vi "Unscale 32 Bit.vi"(8 "error in (no error)":errorcluster, 11 "Data Scaling in":refnum<class "Data Scaling.lvclass">) -> (0 "error out":errorcluster, 3 "Data Scaling out":refnum<class "Data Scaling.lvclass">)   [LabVIEW 2020, in "Unit Tests.lvlib" / "Data Scaling.lvclass"]
uses:
  Data Scaling.lvclass
  Frames & Messages/TypeDefs/Scaling Information.ctl
  <vilib>/addons/_JKI Toolkits/Caraya/classes/Test/Test.lvclass
  <vilib>/addons/_JKI Toolkits/Caraya/classes/Assert/Assert.lvclass
  BCI-1553 API.lvlib
panel:
  out "unscaled number":u64 format="%064b"
  out "base number":u64 format="%064b"
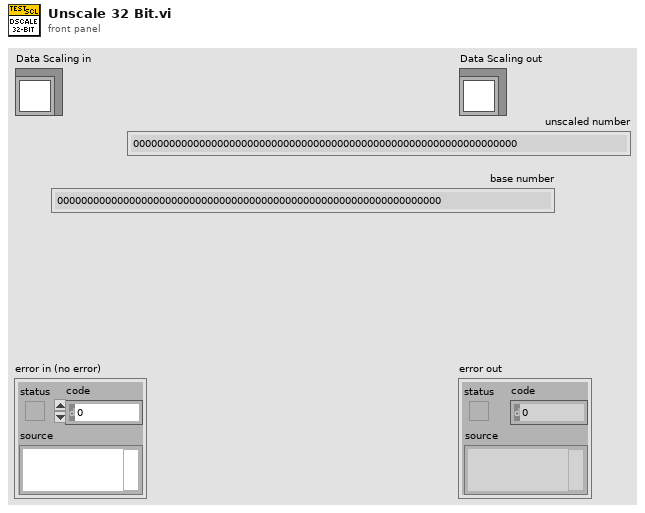
[diagram p1: front panel]
types:
  T1 = typedef "BCI-1553 API.lvlib/Scaling Information.ctl" = cluster{"Bit Offset":i32, "Bit Count":i32, "LSB Resolution":dbl, "2's Complement":bool, "Big Endian":bool, "Sign Bit":bool}
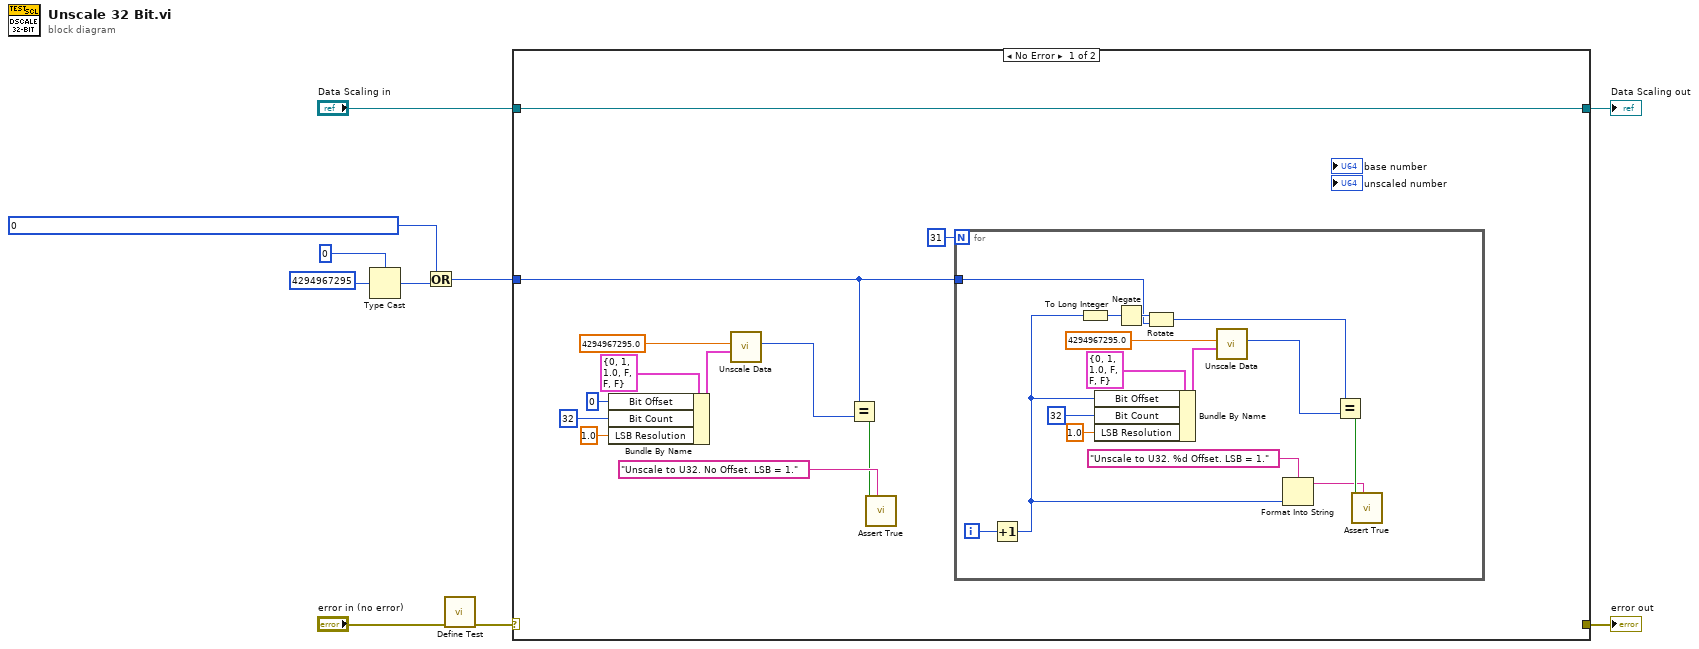
[diagram p0: block diagram]
diagram:
  n1 = Type Cast(type=u64 0 ("x"), x=u32 4294967295 ("unsigned 8bit integer")) -> (*(type *) &x=w4:u64)
  n2 = Or(x=u64 0 ("Raw Value"), y=w4) -> (x .or. y?=w1:u64)
  n3 = call <vilib>:"Define Test.vi"("error in (no error)"="error in (no error)") -> ("error out"=w6:errorcluster)  [unwired: 9 in, 1 out]
  n4 = case shown="No Error" w6 {
    selector: w6 -> [_ w39]
    tunnel: [_ w39] -> w10
    tunnel: [w22 w38] -> w8
    tunnel: "Data Scaling in" -> [w22 w38]
    tunnel: w1 -> [w11 _]
    frame No Error {
      n5 = Bundle By Name(cluster=T1 {"Bit Offset"=0, "Bit Count"=1, "LSB Resolution"=1.0, "2's Complement"=FALSE, "Big Endian"=FALSE, "Sign Bit"=FALSE} ("Scaling Info"), "Bit Offset"=0, "Bit Count"=32, "LSB Resolution"=1.0) -> (w18:T1)
      n6 = call "Unscale Data.vi"("Scaling Info"=w18, "Scaled Value"=4294967295.0 ("y")) -> ("Raw Value"=w20:u64)  [unwired: 8 in, 1 out]
      n7 = Equal?(x=w11, y=w20) -> (x = y?=w16:bool)
      n8 = call <vilib>:"Assert True.vi"("Label"="Unscale to U32. No Offset. LSB = 1.", "True?"=w16) -> ()  [unwired: 8 in, 2 out]
      n9 = for {
        N: 31 -> [_]
        tunnel: w11 -> [w25]
        i -> [w31]
        n10 = Increment(x=w31) -> (x+1=w26:i32)
        n11 = To Long Integer(number=w26) -> (32bit integer=w27:i32)
        n12 = Bundle By Name(cluster=T1 {"Bit Offset"=0, "Bit Count"=1, "LSB Resolution"=1.0, "2's Complement"=FALSE, "Big Endian"=FALSE, "Sign Bit"=FALSE} ("Scaling Info"), "Bit Offset"=w26, "Bit Count"=32, "LSB Resolution"=1.0) -> (w36:T1)
        n13 = Negate(x=w27) -> (-x=w28:i32)
        n14 = Rotate(1:w25, 2:w28) -> (0:w24:u64)
        n15 = call "Unscale Data.vi"("Scaling Info"=w36, "Scaled Value"=4294967295.0 ("y")) -> ("Raw Value"=w23:u64)  [unwired: 8 in, 1 out]
        n16 = Format Into String(format string="Unscale to U32. %d Offset. LSB = 1." ("Label"), w26) -> (resulting string=w29:string)  [unwired: 2 in, 1 out]
        n17 = Equal?(x=w24, y=w23) -> (x = y?=w35:bool)
        n18 = call <vilib>:"Assert True.vi"("Label"=w29, "True?"=w35) -> ()  [unwired: 8 in, 2 out]
      }
    }
    frame Error {
    }
  }
  "error out" <- w10
  "Data Scaling out" <- w8
